vi "UMLEditor RevisionHistory.vi"(0 "localVariables":T1 {"ObjectHotspots"."HotSpot"."y" format="%.2f"; "ObjectHotspots"."HotSpot"."x" format="%.2f"; "NodesBounds"."height" format="%.2f"; "NodesBounds"."width" format="%.2f"; "NodesBounds"."y" format="%.2f"; "NodesBounds"."x" format="%.2f"; "offset"."y" format="%.2f"; "offset"."x" format="%.2f"; "gridSize" format="%.2f"; "dragStartBounds"."height" format="%.2f"; "dragStartBounds"."width" format="%.2f"; "dragStartBounds"."y" format="%.2f"; "dragStartBounds"."x" format="%.2f"; "dragStartPoint"."y" format="%.2f"; "dragStartPoint"."x" format="%.2f"; "rubberBandStart"."y" format="%.2f"; "rubberBandStart"."x" format="%.2f"; "lastMousePoint"."y" format="%.2f"; "lastMousePoint"."x" format="%.2f"; "zoom" format="%.2f"}, 5 "error in (no error)":errorcluster) -> (19 "error out":errorcluster)   [LabVIEW 2014]
doc: "Helpinstructions."
uses:
  <resource>/Framework/Providers/Open_GDS/UML/UMLEditor/UMLEditor LocalVariablesType.ctl
  <resource>/Framework/Providers/Open_GDS/UML/Graphics_class/Graphics.lvclass
  <resource>/Framework/Providers/Open_GDS/UML/Grid_class/Grid.lvclass
  <resource>/Framework/Providers/Open_GDS/UML/AbstractEdge_class/AbstractEdge.lvclass
  <resource>/Framework/Providers/Open_GDS/UML/AbstractNode_class/AbstractNode.lvclass
  <resource>/Framework/Providers/Open_GDS/UML/UMLEditor/UMLEditor statesType.ctl
  <resource>/Framework/Providers/Open_GDS/UML/UMLEditor/UMLEditor tooltype.ctl
  <resource>/Framework/Providers/Open_GDS/UML/UMLEditor/UMLEditor toolsType.ctl
  <resource>/Framework/Providers/Open_GDS/UML/Graph_class/private/diagramType.ctl
  <resource>/Framework/Providers/Open_GDS/UML/Graph_class/Graph.lvclass
  <resource>/Framework/Providers/Open_GDS/UML/General/Point/Point Point2D.ctl
  <resource>/Framework/Providers/Open_GDS/UML/General/Rectangle/Rectangle Rectangle2D.ctl
  <resource>/Framework/Providers/Open_GDS/UML/UMLEditor/UMLEditor ExportType.ctl
  <resource>/Framework/Providers/Open_GDS/UML/UMLEditor/UMLEditor FlattenCommandType.ctl
  <resource>/Framework/Providers/Open_GDS/UML/UMLEditor/UMLEditor ExecuteCommandType.ctl
  <resource>/Framework/Providers/Open_GDS/UML/ContextHelp/ContextHelp_EventType.ctl
  <resource>/Framework/Providers/Open_GDS/UML/UMLEditor/UMLEditor_HotSpotData.ctl
  <resource>/Framework/Providers/Open_GDS/UML/UMLEditor/UMLEditor_HotSpotType.ctl
panel:
  out "rev":string
  in  "Ok":bool
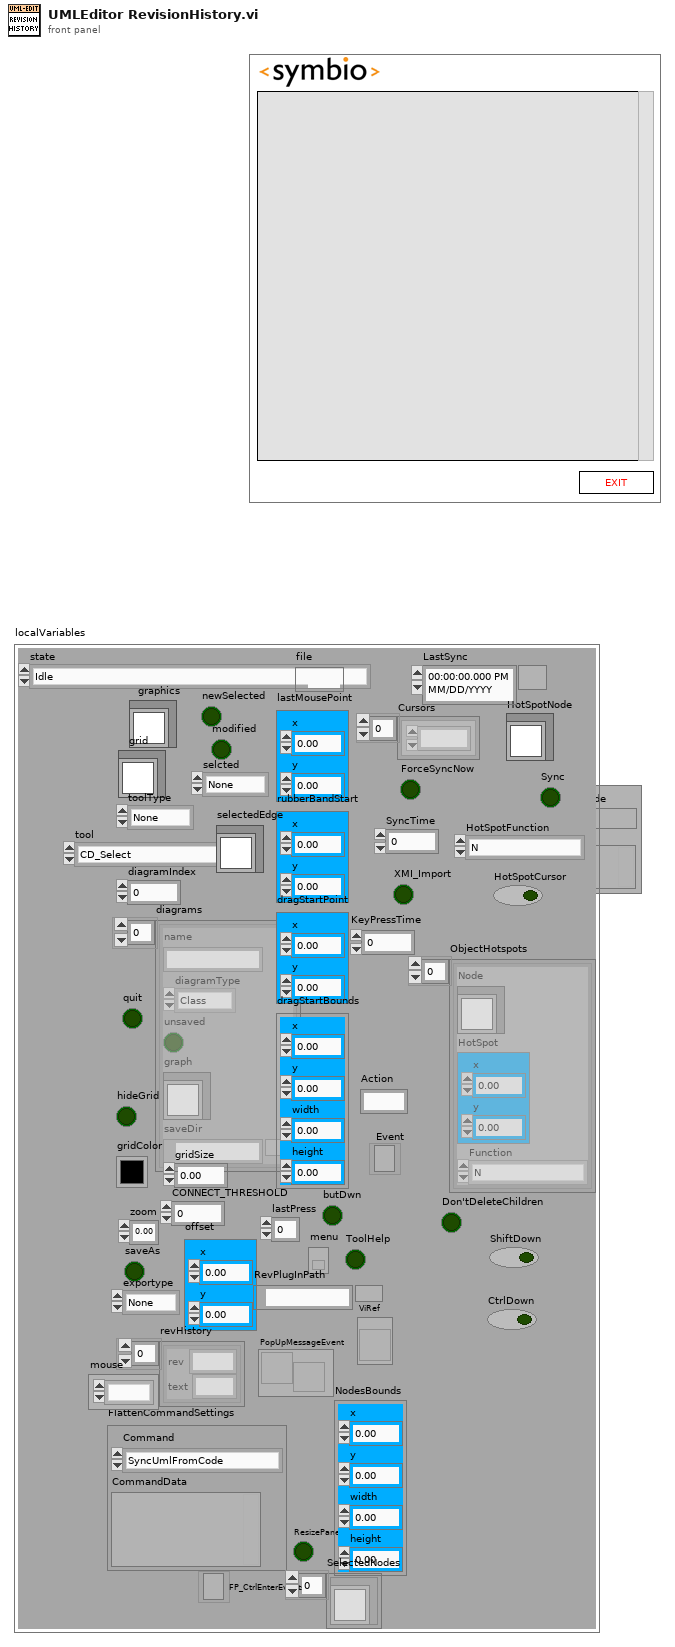
[diagram p1: front panel]
types:
  T1 = typedef "UMLEditor LocalVariablesType.ctl" = cluster{"state":T2, "graphics":refnum<class "Graphics.lvclass">, "grid":refnum<class "Grid.lvclass">, "toolType":T3, "tool":T4, "diagramIndex":i32, "diagrams":cluster{"name":string, "diagramType":T5, "unsaved":bool, "graph":refnum<class "Graph.lvclass">, "saveDir":path}[], "zoom":dbl, "hideGrid":bool, "lastMousePoint":T6, "rubberBandStart":T6, "dragStartPoint":T6, "dragStartBounds":T7, "gridColor":u32, "gridSize":dbl, "CONNECT_THRESHOLD":i32, "selcted":T3, "selectedEdge":refnum<class "AbstractEdge.lvclass">, "butDwn":bool, "lastPress":u32, "modified":bool, "offset":T6, "menu":refnum<k9>, "file":path, "saveAs":bool, "newSelected":bool, "exportype":T8, "quit":bool, "revHistory":cluster{"rev":string, "text":string}[], "FlattenCommandSettings":T9, "PopUpMessageEvent":T11, "ResizePanelInProgress":bool, "NodesBounds":T7, "ToolHelp":bool, "ViRef":refnum<vi>, "FP_CtrlEnterEvents":refnum<event-registration>, "SelectedNodes":refnum<class "AbstractNode.lvclass">[], "mouse":refnum<k1>, "RevPlugInPath":path, "Event":refnum<event-registration>, "Action":string, "KeyPressTime":u32, "Cursors":refnum<k1>[], "ObjectHotspots":T12[], "HotSpotCursor":bool, "HotSpotFunction":T13, "Don'tDeleteChildren":bool, "ShiftDown":bool, "CtrlDown":bool, "HotSpotNode":refnum<class "AbstractNode.lvclass">, "Sync":bool, "SyncTime":u32, "ForceSyncNow":bool, "LastSync":timestamp, "XMI_Import":bool}
  T2 = typedef "UMLEditor statesType.ctl" = enum16{"Idle", "CheckLicense", "revHistory", "Init", "Init2", "EditSelected", "RemoveSelected", "PaintComponent", "ChangeZoom", "ChangeGridSize", "Open", "Close", "Save", "ExportPicture", "Export", "Repaint", "Error", "Exit", "QUIT", "CreateScript", "ExecuteScript", "ClassReversedEngineering", "PlugInReverseEngineering", "StateReversedEngineering", "AutoPlace", "ExecuteCommand", "OpenClass", "SyncAll", "StraightenAssociation", "Copy", "Paste", "AddNodeFromProjectTree", "AddNodeFromProjectTree+SyncAll", "PanAndRepaint", "Init3", "CopyPaste", "ApplyDesignPattern", "AnalyseViInStateDiagram", "AutoSync"}
  T3 = typedef "UMLEditor tooltype.ctl" = enum16{"None", "Node", "Edge"}
  T4 = typedef "UMLEditor toolsType.ctl" = enum16{"CD_Select", "CD_Class", "CD_Interface", "CD_Package", "CD_Note", "CD_Dependency", "CD_Inheritance", "CD_InterfaceImp", "CD_Association", "CD_Aggregation", "CD_Composite", "CD_NoteConn", "SQD_Select", "SQD_Object", "SQD_ActionBar", "SQD_Note", "SQD_Call", "SQD_NoteConn", "UD_Select", "UD_System", "UD_Actor", "UD_UseCase", "UD_Note", "UD_Assoiciation", "UD_Generalization", "UD_GeneralizationIncludes", "UD_GeneralizationExtends", "UD_Realization", "UD_Relationship", "UD_NoteEdge", "STD_Select", "STD_State", "STD_InitailState", "STD_FinalState", "STD_ChoiseState", "STD_StateTransation", "STD_Note", "STD_NoteEdge"}
  T5 = typedef "Graph.lvclass/diagramType.ctl" = enum16{"None", "Class", "Sequency", "State", "UseCase"}
  T6 = typedef "Point Point2D.ctl" = cluster{"x":dbl, "y":dbl}
  T7 = typedef "Rectangle Rectangle2D.ctl" = cluster{"x":dbl, "y":dbl, "width":dbl, "height":dbl}
  T8 = typedef "UMLEditor ExportType.ctl" = enum16{"None", "Printer", "png", "jpg", "roseUML"}
  T9 = typedef "UMLEditor FlattenCommandType.ctl" = cluster{"Command":T10, "CommandData":variant}
  T10 = typedef "UMLEditor ExecuteCommandType.ctl" = enum16{"SyncUmlFromCode", "SyncCodeFromUML", "OpenClass", "OpenFile", "CreateClass", "CreateVI", "OpenClassAttribute", "LocateInProject"}
  T11 = typedef "ContextHelp_EventType.ctl" = refnum<user-event>
  T12 = typedef "UMLEditor_HotSpotData.ctl" = cluster{"Node":refnum<class "AbstractNode.lvclass">, "HotSpot":T6, "Function":T13}
  T13 = typedef "UMLEditor_HotSpotType.ctl" = enum16{"N", "NE", "E", "SE", "S", "SW", "W", "NW", "Expand", "Collaps"}
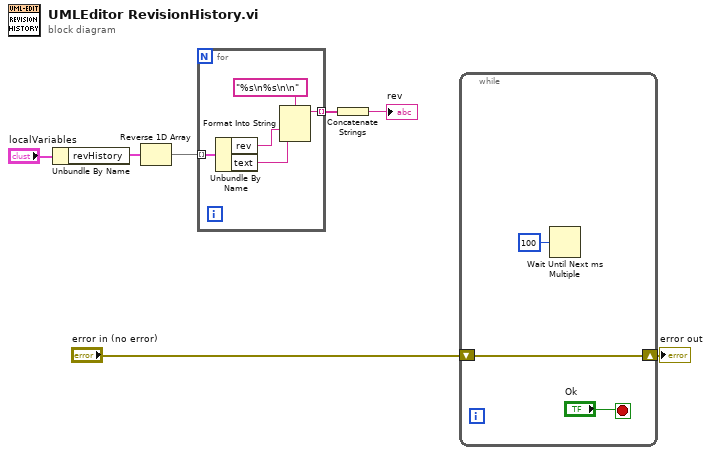
[diagram p0: block diagram]
diagram:
  n1 = Unbundle By Name("localVariables") -> ("revHistory"=w4:cluster{"rev":string, "text":string}[])
  n2 = Reverse 1D Array(array=w4) -> (reversed array=w1:cluster{"rev":string, "text":string}[])
  n3 = for {
    tunnel: w1 -> [w12] mode=indexing
    tunnel: [w8] -> w3 mode=indexing
    n4 = Unbundle By Name(w12) -> ("rev"=w10:string, "text"=w9:string)
    n5 = Format Into String(format string="%s\n%s\n\n", w10, w9) -> (resulting string=w8:string)  [unwired: 2 in, 1 out]
  }
  n6 = Concatenate Strings(w3) -> (→"rev":string)
  n7 = while {
    shift-left: "error in (no error)" -> [w13]
    shift-right: [w13] -> w7
    stop <- "Ok" stop-if-true
    n8 = Wait Until Next ms Multiple(millisecond multiple=u32 100 ("milliseconds to wait")) -> ()  [unwired: 1 out]
  }
  "error out" <- w7
